vi "Main_rownolegle.vi"() -> ()   [LabVIEW 2013]
doc: "Use this template to build a producer/consumer design pattern. Use this template when you need to execute a process, such as data analysis, when a data source, such as a triggered acquisition, produces data at an uneven rate and you need to execute the process when the data becomes available."
uses:
  inne pliki/Params.ctl
  inne pliki/Stany.ctl
  inne pliki/Data.ctl
  inne pliki/Akcje rownolegle FVG.ctl
panel:
  out "Czas":string
  in  "Zakres uśredniania (5)":i32=5
  in  "Temp limits":T1={"Max (25)"=25.0, "Min (0)"=0.0}
  out "Waveform Chart":T2(graph)
  out "Warning text":string
  out "Warning":bool
  in  "stop":bool
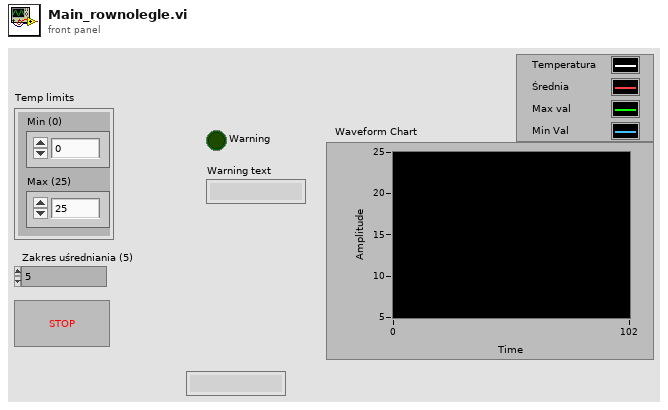
[diagram p1: front panel]
types:
  T1 = typedef "Params.ctl" = cluster{"Max (25)":dbl, "Min (0)":dbl}
  T2 = cluster{"Temperatura":dbl, "Średnia":dbl, "Max (25)":dbl, "Min (0)":dbl}
  T3 = typedef "Data.ctl" = cluster{"Temperatura":dbl, "Średnia":dbl, "Warning":bool, "Warning text ":string, "Temp limits":T1, "Temp Array":dbl[], "Sternia Array":dbl[]}
  T4 = typedef "Stany.ctl" = enum16{"Config", "IDLE", "Measure", "Analyze", "Display", "STOP", "Save"}
  T5 = typedef "Akcje rownolegle FVG.ctl" = enum16{"SET", "GET"}
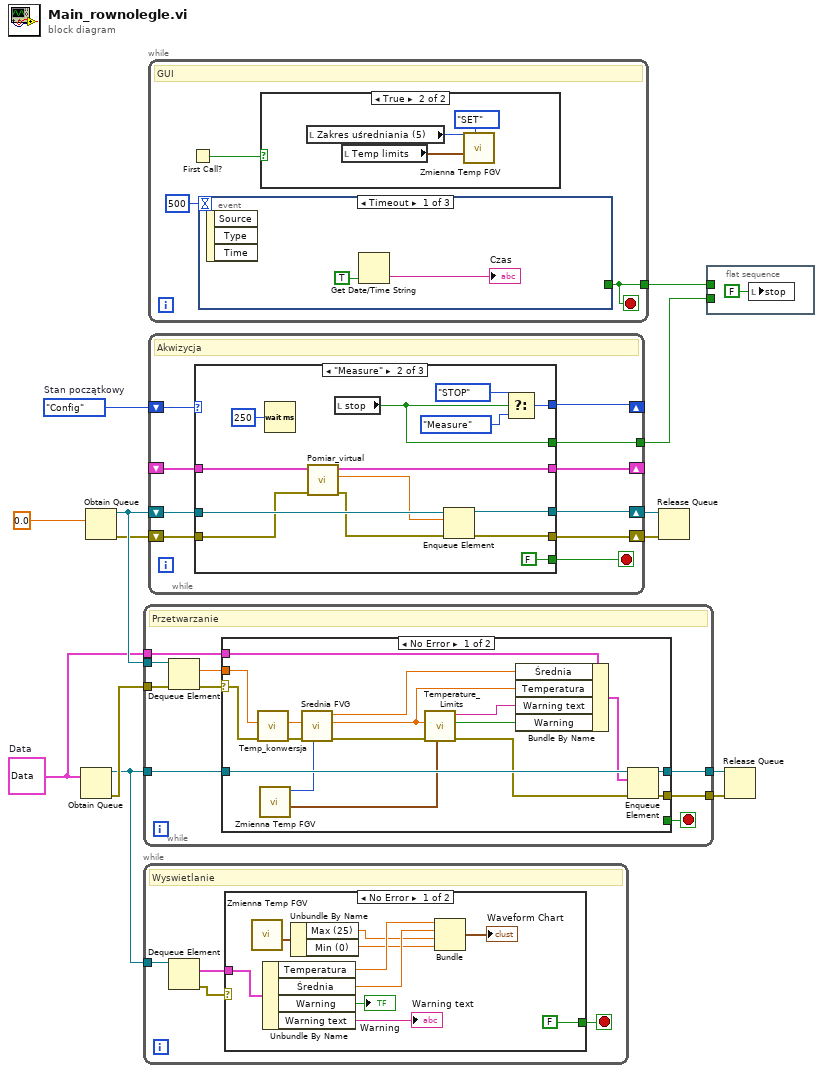
[diagram p0: block diagram]
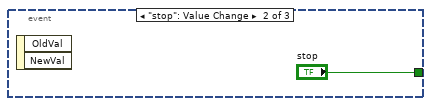
[diagram p3: hidden frame]
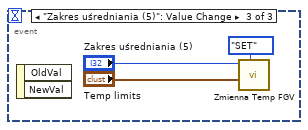
[diagram p4: hidden frame]
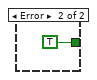
[diagram p5: hidden frame]
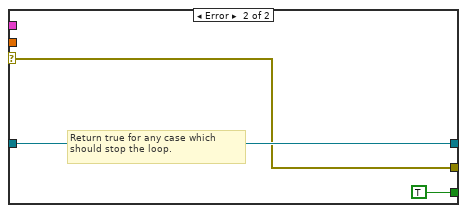
[diagram p6: hidden frame]
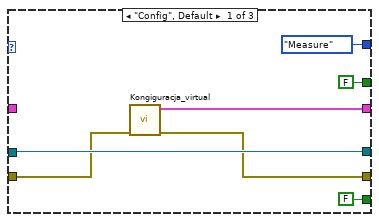
[diagram p7: hidden frame]
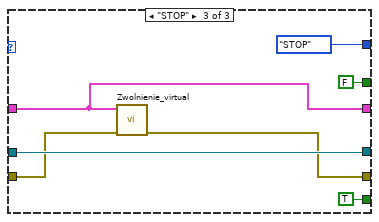
[diagram p8: hidden frame]
diagram:
  w3 = T3 {"Temperatura"=0.0, "Średnia"=0.0, "Warning"=FALSE, "Warning text "="", "Temp limits"={"Max (25)"=25.0, "Min (0)"=0.0}, "Temp Array"=[], "Sternia Array"=[]}  # Data
  w9 = Stany."Config"  # Stan początkowy
  n1 = Obtain Queue(element data type=w3) -> (queue out=w4:refnum<queue>, error out=w7:errorcluster)  [unwired: 4 in, 1 out]
  n2 = Obtain Queue(element data type=0.0) -> (queue out=w13:refnum<queue>, error out=w12:errorcluster)  [unwired: 4 in, 1 out]
  n3 = while {
    tunnel: w13 -> [w22]
    tunnel: w4 -> [w18]
    tunnel: w7 -> [w17]
    tunnel: [w16] -> w6
    tunnel: [w15] -> w5
    tunnel: w3 -> [w14]
    stop <- w19 stop-if-true
    # "Przetwarzanie"
    n4 = Dequeue Element(queue=w22, error in (no error)=w17) -> (element=w20:dbl, error out=w21:errorcluster)  [unwired: 1 in, 2 out]
    n5 = case shown="No Error" w21 {
      selector: w21 -> [w36 w40]
      tunnel: w20 -> [w37 _]
      tunnel: [_ TRUE] -> w19
      tunnel: w18 -> [w35 w41]
      tunnel: [w32 w41] -> w16
      tunnel: [w31 w40] -> w15
      tunnel: w14 -> [w25 _]
      frame No Error {
        n6 = call "Temp_konwersja.vi"("error in (no error)"=w36, "Temp in"=w37) -> ("error out"=w38:errorcluster, "Temp out"=w39:dbl)  [unwired: 8 in]
        n7 = call "Zmienna Temp FGV.vi"() -> ("Temp limits out"=w23:T1, "Zakres out"=w24:i32)  [unwired: 9 in, 1 out]
        n8 = call "Srednia FVG.vi"("Zakres (5)"=w24, "error in (no error)"=w38, "temperatura in"=w39) -> ("error out"=w34:errorcluster, "temperatura out"=w29:dbl, "średnia out"=w30:dbl)  [unwired: 6 in]
        n9 = call "Temperature_Limits.vi"("Temp limits"=w23, "error in (no error)"=w34, "TEMP"=w29) -> ("error out"=w33:errorcluster, "Warning"=w27:bool, "Warning Text"=w28:string)  [unwired: 6 in]
        n10 = Bundle By Name(cluster=w25, "Średnia"=w30, "Temperatura"=w29, "Warning text"=w28, "Warning"=w27) -> (w26:T3)
        n11 = Enqueue Element(queue=w35, element=w26, error in (no error)=w33) -> (queue out=w32:refnum<queue>, error out=w31:errorcluster)  [unwired: 1 in, 1 out]
      }
      frame Error {
        # "Return true for any case which should stop the loop."
      }
    }
  }
  n12 = while {
    tunnel: w4 -> [w46]
    stop <- w43 stop-if-true
    # "Wyswietlanie"
    n13 = Dequeue Element(queue=w46) -> (element=w45:T3, error out=w44:errorcluster)  [unwired: 2 in, 2 out]
    n14 = case shown="No Error" w44 {
      tunnel: w45 -> [w56 _]
      tunnel: [FALSE TRUE] -> w43
      frame No Error {
        n15 = call "Zmienna Temp FGV.vi"() -> ("Temp limits out"=w49:T1)  [unwired: 9 in, 2 out]
        n16 = Unbundle By Name(w56) -> ("Temperatura"=w52:dbl, "Średnia"=w51:dbl, "Warning"=→"Warning":bool, "Warning text"=→"Warning text":string)
        n17 = Unbundle By Name(w49) -> ("Max (25)"=w48:dbl, "Min (0)"=w47:dbl)
        n18 = Bundle("Temperatura"=w52, "Średnia"=w51, "Max (25)"=w48, "Min (0)"=w47) -> (→"Waveform Chart":T2)  [unwired: 1 in]
      }
      frame Error {
      }
    }
  }
  n19 = while {
    tunnel: [w60] -> w2
    stop <- w60 stop-if-true
    # "GUI"
    n20 = First Call?() -> (First Call?: T/F=w59:bool)
    n21 = event shown="[0] Timeout" {
      selector: _ -> [_ _ _]
      dyn-events: _ -> [_ _ _]
      timeout: 500 -> [_ _ _]
      tunnel: [_ "stop" _] -> w60
      event Timeout {
        n22 = event-data() -> ()  [unwired: 1 in, 3 out]
        n23 = Get Date/Time String(want seconds? (F)=TRUE) -> (time string=→"Czas":string)  [unwired: 2 in, 1 out]
      }
      event "stop": Value Change {
        n24 = event-data() -> ()  [unwired: 1 in, 2 out]
      }
      event "Zakres uśredniania (5)": Value Change {
        n25 = event-data() -> ()  [unwired: 1 in, 2 out]
        n26 = call "Zmienna Temp FGV.vi"("Akcje (GET)"=Akcje_rownolegle_FVG."SET", "Temp limits in"="Temp limits", "Zakres in"="Zakres uśredniania (5)") -> ()  [unwired: 6 in, 3 out]
      }
    }
    n27 = case shown="True" w59 {
      frame False {
      }
      frame True {
        n28 = local read "Zakres uśredniania (5)"() -> (w61:i32)
        n29 = local read "Temp limits"() -> (w62:T1)
        n30 = call "Zmienna Temp FGV.vi"("Akcje (GET)"=Akcje_rownolegle_FVG."SET", "Temp limits in"=w62, "Zakres in"=w61) -> ()  [unwired: 6 in, 3 out]
      }
    }
  }
  n31 = while {
    shift-right: [w74] -> w10
    shift-left: w12 -> [w73]
    shift-right: [w75] -> w11
    shift-left: w13 -> [w76]
    shift-right: [w78] -> _
    shift-left: w9 -> [w79]
    shift-right: [w72] -> _
    shift-left: _ -> [w71]
    tunnel: [w70] -> w1
    stop <- w77 stop-if-true
    # "Akwizycja"
    n32 = case shown="\"Measure\"" w79 {
      tunnel: [Stany."Measure" ("Stan") w98 Stany."STOP" ("Stan")] -> w78
      tunnel: [FALSE FALSE TRUE] -> w77
      tunnel: w76 -> [w84 w96 w105]
      tunnel: [w84 w95 w105] -> w75
      tunnel: [w81 w91 w103] -> w74
      tunnel: w73 -> [w82 w89 w104]
      tunnel: [w83 w93 w102] -> w72
      tunnel: w71 -> [_ w94 w102]
      tunnel: [FALSE ("stop") w87 FALSE ("stop")] -> w70
      frame "Config", Default {
        n33 = call "Kongiguracja_virtual.vi"("error in (no error)"=w82) -> ("error out"=w81:errorcluster, "Reference out"=w83:cluster{"Numeric":dbl, "Boolean":bool})  [unwired: 9 in]
      }
      frame "Measure" {
        n34 = Wait (ms)(milliseconds to wait=u32 250) -> ()  [unwired: 1 out]
        n35 = call "Pomiar_virtual.vi"("error in (no error)"=w89, "Reference in"=w94) -> ("error out"=w90:errorcluster, "out"=w92:dbl, "Reference out"=w93:cluster{"Numeric":dbl, "Boolean":bool})  [unwired: 7 in]
        n36 = local read "stop"() -> (w87:bool)
        n37 = Enqueue Element(queue=w96, element=w92, error in (no error)=w90) -> (queue out=w95:refnum<queue>, error out=w91:errorcluster)  [unwired: 1 in, 1 out]
        n38 = Select(t=Stany."STOP" ("Stan"), s=w87, f=Stany."Measure" ("Stan")) -> (s? t:f=w98:T4)
      }
      frame "STOP" {
        n39 = call "Zwolnienie_virtual.vi"("error in (no error)"=w104, "Reference in"=w102) -> ("error out"=w103:errorcluster)  [unwired: 9 in]
      }
    }
  }
  n40 = Release Queue(queue=w11, error in (no error)=w10) -> ()  [unwired: 1 in, 3 out]
  n41 = flat-sequence {
    tunnel: w2 -> [_]
    tunnel: w1 -> [_]
    frame #0 {
      n42 = local write "stop"(FALSE ("stop")) -> ()
    }
  }
  n43 = Release Queue(queue=w6, error in (no error)=w5) -> ()  [unwired: 1 in, 3 out]
